vi "Match Literal Prefix.vi"(4 "case matching (sensitive)":T1=enum."system", 6 "offset (0)":i32, 7 "string":string, 8 "literal prefix":string) -> (0 "offset past match":i32, 1 "found substring":bool, 2 "after substring":string, 3 "match substring":string, 5 "before substring":string)   [LabVIEW 2009, in "Tools_String.lvlib"]
uses:
  Tools_String.lvlib
  Case Matching.ctl
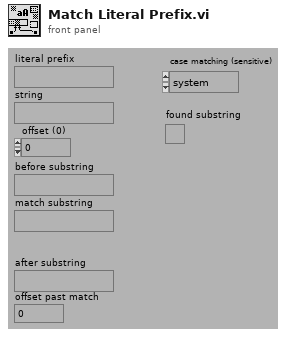
[diagram p1: front panel]
types:
  T1 = typedef "Tools_String.lvlib/Case Matching.ctl" = enum16{"a != A", "a == A", "system"}
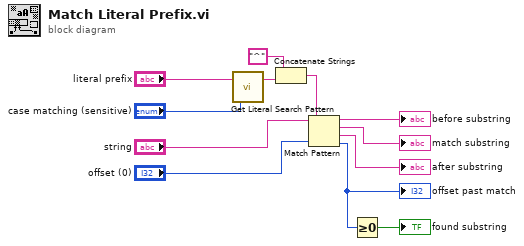
[diagram p0: block diagram]
diagram:
  n1 = call "Get Literal Search Pattern.vi"("case matching (sensitive)"="case matching (sensitive)", "literal string"="literal prefix") -> ("regular expression"=w2:string)  [unwired: 1 out]
  n2 = Concatenate Strings("^", w2) -> (w4:string)
  n3 = Match Pattern(string="string", regular expression=w4, offset (0)="offset (0)") -> (before substring=→"before substring":string, match substring=→"match substring":string, after substring=→"after substring":string, offset past match=w6:i32)
  "offset past match" <- w6
  n4 = Greater Or Equal To 0?(x=w6) -> (x >= 0?=→"found substring":bool)
